vi "Flush Queues.vi"(8 "error in":errorcluster, 11 "server in":refnum<class "RT FlexRIO Server TCP.lvclass">) -> (0 "error out":errorcluster, 3 "server out":refnum<class "RT FlexRIO Server TCP.lvclass">)   [LabVIEW 2017, in "RT FlexRIO Server TCP.lvclass"]
uses:
  RT FlexRIO Server TCP.lvclass
  Properties/IncomingQueue_GET.vi
  Properties/OutgoingQueue_GET.vi
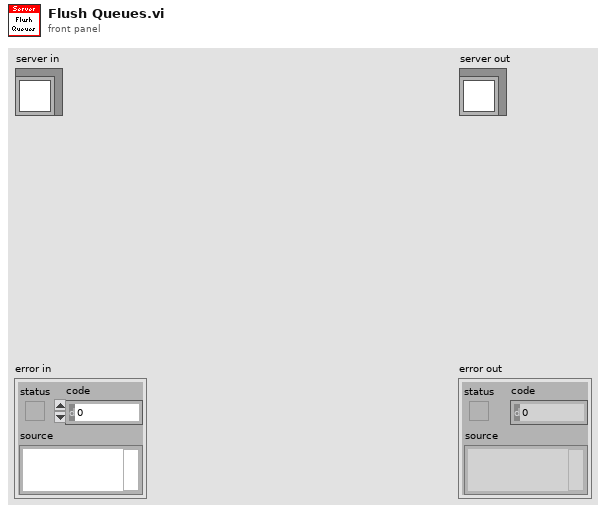
[diagram p1: front panel]
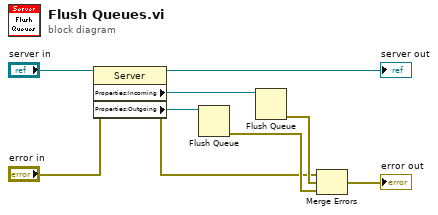
[diagram p0: block diagram]
diagram:
  n1 = property class="Server"(reference="server in", error in="error in") -> (reference out=→"server out":refnum<class "RT FlexRIO Server TCP.lvclass">, error out=w1:errorcluster, "Properties:Incoming"=w7:refnum<queue>, "Properties:Outgoing"=w8:refnum<queue>)
  n2 = Flush Queue(queue=w8) -> (error out=w5:errorcluster)  [unwired: 1 in, 2 out]
  n3 = Flush Queue(queue=w7) -> (error out=w6:errorcluster)  [unwired: 1 in, 2 out]
  n4 = Merge Errors(w1, w6, w5) -> (→"error out":errorcluster)
